vi "Add Line Feed.vi"(4 "Command string":string) -> (1 "Concatenated string":string)   [LabVIEW 2025, in "Chroma 19052.lvlib"]
uses:
  <instrlib>/Chroma 19052/Chroma 19052.lvlib
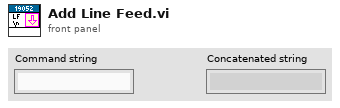
[diagram p1: front panel]
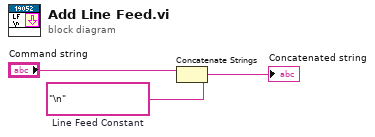
[diagram p0: block diagram]
diagram:
  w3 = "\n"  # Line Feed Constant
  n1 = Concatenate Strings("Command string", w3) -> (→"Concatenated string":string)
